vi "OptAcq332Tlog.vi"(0 "Configurations":string[](array[string]), 1 "ConfigsVal In":u16[](array[numeric]), 2 "XY Graph Ref 2":refnum<vi>, 3 "TracerOpts In":u8[](array[numeric]), 4 "AcqenCours":bool caption="Acquisition en Cours", 5 "error in":errorcluster, 6 "VISA Rsrc":refnum<visa-resource-name>="GPIB0::12::INSTR" caption="Nom de la ressource VISA", 7 "Activées In":bool[](array[boolean]) caption="Entrés Activées In") -> (10 "TablesConv":u16[](array[numeric]) caption="No Courbe de conversion" max=60 step=1, 11 "Scan list Out":string[](array[string]), 12 "TracerCourbe":bool[](array[boolean]), 13 "OneChangeAppl":bool caption="Changements Appliqués out", 14 "ConfigsChoisi":string[](array[string]), 15 "ConfigsVal Out":u16[](array[numeric]), 16 "Activées":bool[](array[boolean]) caption="Entrés Activées Out", 17 "TracerOpts Out":u8[](array[numeric]), 18 "Entête":string, 19 "error out":errorcluster)   [LabVIEW 2010]
doc: "Ce Vi permet d'activer et d'attribuer une configuration à chaque entrée du contrôlleur de température. Il permet aussi de choisir les options de traçage des données de température, de niveau d'hélium et de chaufage."
panel:
  in  "Forcer":bool caption="Forcer la mise à jour"
  in  "Chauffage":bool=TRUE caption="Tracer le Chauffage"
  out "Changé":bool[](array[boolean]) caption="Entrés Changé"
  in  "Activé B":bool=TRUE caption="Activée"
  in  "Activé A":bool=TRUE caption="Activée"
  in  "NiveauHe":bool=TRUE caption="Tracer le niveau d'hélium"
  out "LastChangeAppl":bool caption="Changements Appliqués"
  in  "TracerOpt B":u8(ring)=2 caption="Données à Tracer" items=["Unités Capteurs", "Unité Labview", "Ne Pas Tracer"]
  in  "Config B":u16(ring) caption="Nom de la Configuration" items=["Default", "Pompe à adsorption", "Pot à 1K", "Pot à He3", "Échantillon", "Cleaver"]
  in  "TracerOpt A":u8(ring)=2 caption="Données à Tracer" items=["Unités Capteurs", "Unité Labview", "Ne Pas Tracer"]
  in  "Apply":bool
  in  "OK":bool
  in  "Config A":u16(ring) caption="Nom de la Configuration" items=["Default", "Pompe à adsorption", "Pot à 1K", "Pot à He3", "Échantillon", "Cleaver"]
  # "Paramètres d'acquisition"
  # "Entrée A"
  # "Entrée B"
  # "Variables internes"
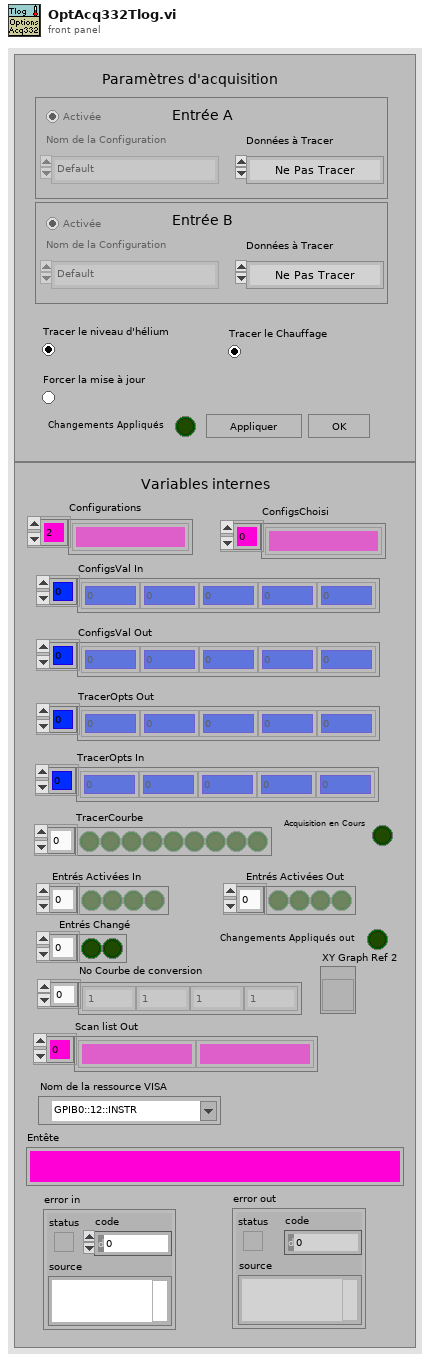
[diagram p1: front panel]
types:
  T1 = enum32{"Invalid", "Standard", "Closed", "Hidden", "Minimized", "Maximized"}
  T2 = typedef "InConfigPar332.ctl" = cluster{"TableTC":u16, "TableConv":u16, "Compensation":u16, "Type":u16}
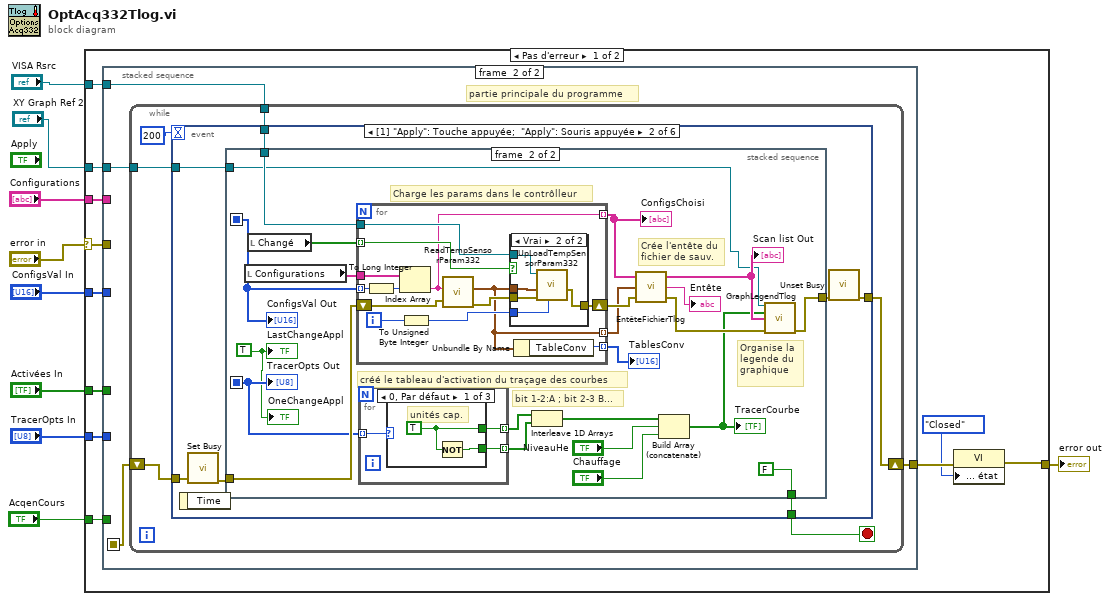
[diagram p0: block diagram]
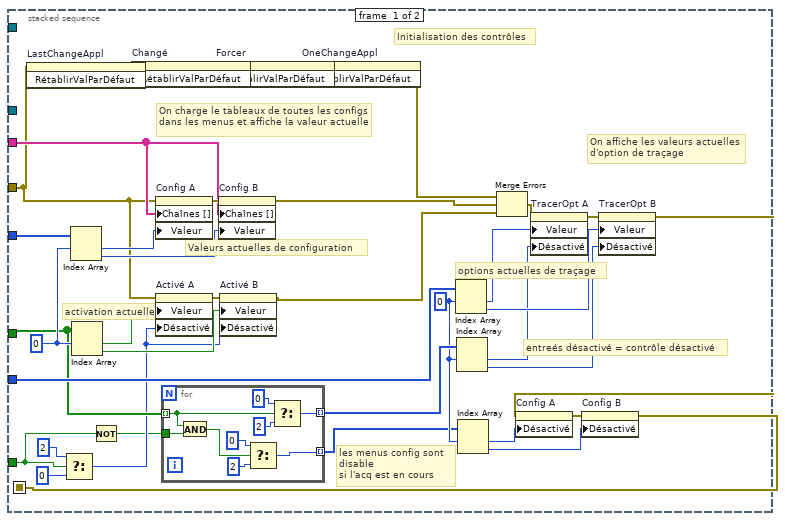
[diagram p2: hidden frame]
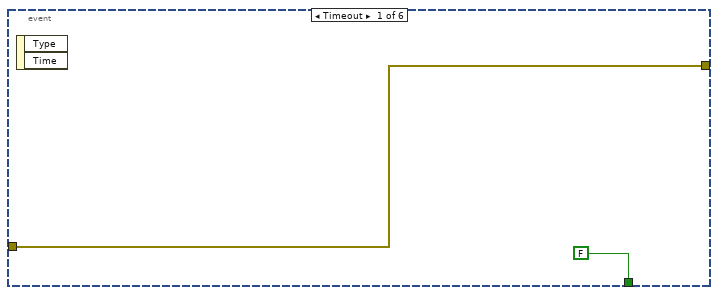
[diagram p3: hidden frame]
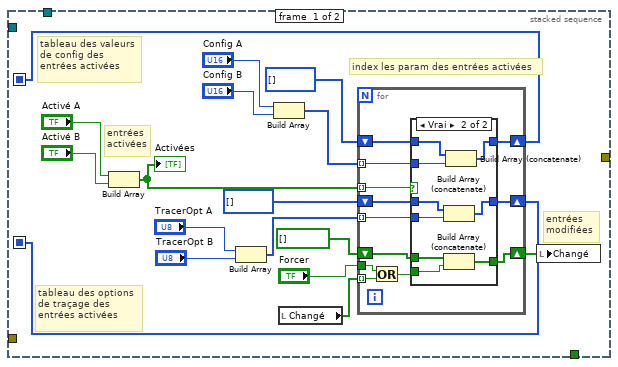
[diagram p4: hidden frame]
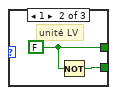
[diagram p6: hidden frame]
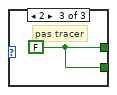
[diagram p7: hidden frame]
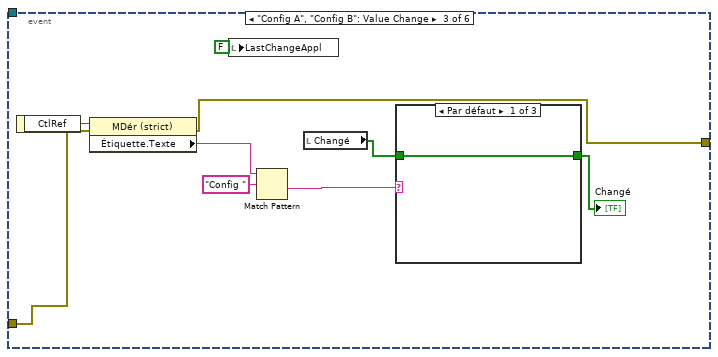
[diagram p9: hidden frame]
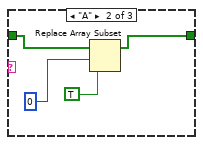
[diagram p10: hidden frame]
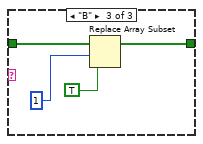
[diagram p11: hidden frame]
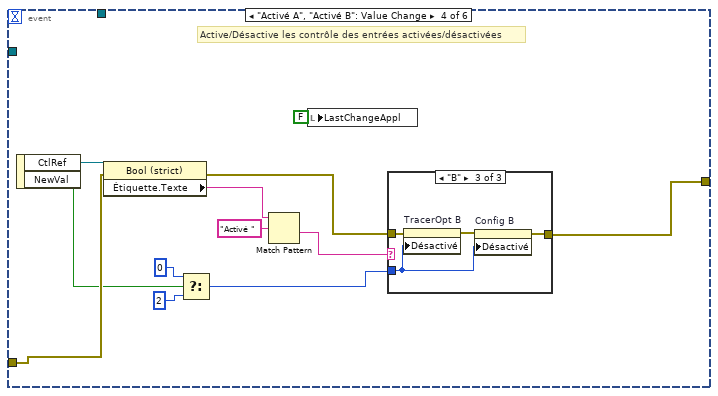
[diagram p12: hidden frame]
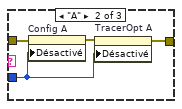
[diagram p14: hidden frame]
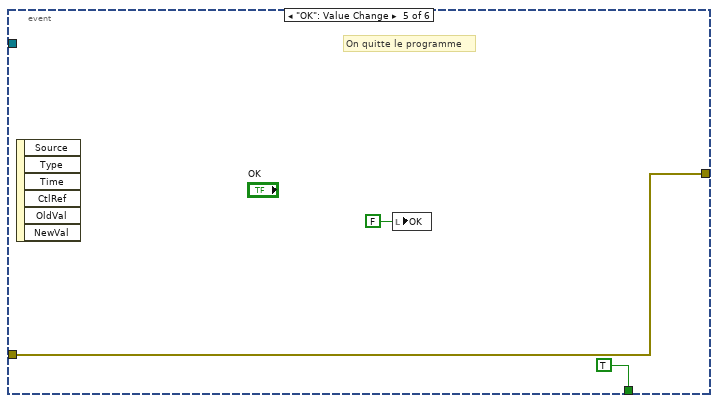
[diagram p15: hidden frame]
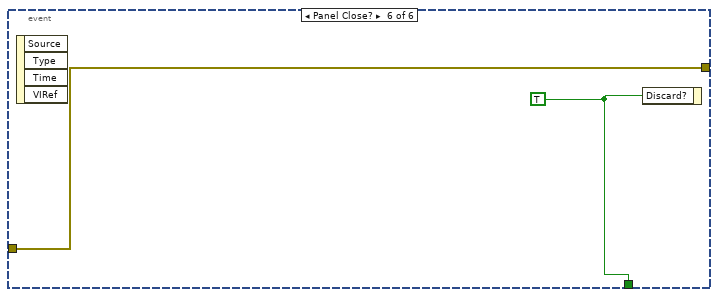
[diagram p16: hidden frame]
diagram:
  n1 = case shown="Pas d'erreur" "error in" {
    selector: "error in" -> [w19 w221]
    tunnel: [w11 w221] -> w9
    tunnel: "Configurations" -> [w20 _]
    tunnel: "ConfigsVal In" -> [w18 _]
    tunnel: "TracerOpts In" -> [w17 _]
    tunnel: "AcqenCours" -> [w16 _]
    tunnel: "Activées In" -> [w15 _]
    tunnel: "XY Graph Ref 2" -> [w14 _]
    tunnel: "VISA Rsrc" -> [w13 _]
    frame No Error {
      n2 = stacked-sequence {
        seq-local: [w21 _] -> [_ w70]
        tunnel: w20 -> [w56 _]
        tunnel: w19 -> [w42 _]
        tunnel: w18 -> [w49 _]
        tunnel: w17 -> [w53 _]
        tunnel: [_ w69] -> w12
        tunnel: w16 -> [w35 _]
        tunnel: w15 -> [w40 _]
        tunnel: w14 -> [_ w68]
        tunnel: w13 -> [_ w67]
        frame #0 {
          w33 = 0 ("index")
          w45 = 0 ("index")
          # "les menus config sont disable\nsi l'acq est en cours"
          # "entreés désactivé = contrôle désactivé"
          # "activation actuelle"
          # "Valeurs actuelles de configuration"
          # "options actuelles de traçage"
          # "On affiche les valeurs actuelles d'option de traçage"
          # "On charge le tableaux de toutes les configs dans les menus et affiche la valeur actuelle"
          # "Initialisation des contrôles"
          n3 = invoke on="LastChangeAppl" class="Bool (strict)" method="RétablirValParDéfaut"(error in=w42) -> (error out=w28:errorcluster)  [unwired: 2 in, 2 out]
          n4 = Select(t=u8 2 ("f"), s=w35, f=u8 0) -> (s? t:f=w39:u8)
          n5 = Index Array(array=w49, index #1=w45) -> (element #1=w55:u16, element #2=w54:u16)  [unwired: 1 in]
          n6 = Index Array(array=w40, index #1=w45) -> (element #1=w44:bool, element #2=w43:bool)  [unwired: 1 in]
          n7 = Not(x=w35) -> (.not. x?=w29:bool)
          n8 = invoke on="Changé" class="Array (strict)" method="RétablirValParDéfaut"(error in=w28) -> (error out=w27:errorcluster)  [unwired: 2 in, 2 out]
          n9 = property on="Config A" class="MDér (strict)"(error in=w42, "Chaînes []"=w56, "Valeur"=w55) -> (error out=w57:errorcluster)  [unwired: 1 in, 1 out]
          n10 = property on="Activé A" class="Bool (strict)"(error in=w42, "Valeur"=w44, "Désactivé"=w39) -> (error out=w41:errorcluster)  [unwired: 1 in, 1 out]
          n11 = for {
            tunnel: w40 -> [w60] mode=indexing
            tunnel: [w62] -> w38 mode=indexing
            tunnel: w29 -> [w59]
            tunnel: [w61] -> w30 mode=indexing
            n12 = And(x=w60, y=w59) -> (x .and. y?=w58:bool)
            n13 = Select(t=u8 0 ("f"), s=w58, f=u8 2) -> (s? t:f=w61:u8)
            n14 = Select(t=u8 0 ("f"), s=w60, f=u8 2) -> (s? t:f=w62:u8)
          }
          n15 = invoke on="Forcer" class="Boolean (strict)" method="RétablirValParDéfaut"(error in=w27) -> (error out=w26:errorcluster)  [unwired: 2 in, 2 out]
          n16 = property on="Config B" class="MDér (strict)"(error in=w57, "Chaînes []"=w56, "Valeur"=w54) -> (error out=w23:errorcluster)  [unwired: 1 in, 1 out]
          n17 = property on="Activé B" class="Bool (strict)"(error in=w41, "Valeur"=w43, "Désactivé"=w39) -> (error out=w24:errorcluster)  [unwired: 1 in, 1 out]
          n18 = invoke on="OneChangeAppl" class="Boolean (strict)" method="RétablirValParDéfaut"(error in=w26) -> (error out=w25:errorcluster)  [unwired: 2 in, 2 out]
          n19 = Index Array(array=w53, index #1=w33) -> (element #1=w51:u8, element #2=w50:u8)  [unwired: 1 in]
          n20 = Index Array(array=w38, index #1=w33) -> (element #1=w37:u8, element #2=w36:u8)  [unwired: 1 in]
          n21 = Index Array(array=w30, index #1=w33) -> (element #1=w32:u8, element #2=w31:u8)  [unwired: 1 in]
          n22 = Merge Errors(w25, w23, w24) -> (w47:errorcluster)
          n23 = property on="TracerOpt A" class="MDér (strict)"(error in=w47, "Valeur"=w51, "Désactivé"=w37) -> (error out=w52:errorcluster)  [unwired: 1 in, 1 out]
          n24 = property on="TracerOpt B" class="MDér (strict)"(error in=w52, "Valeur"=w50, "Désactivé"=w36) -> (error out=w22:errorcluster)  [unwired: 1 in, 1 out]
          n25 = property on="Config A" class="MDér (strict)"(error in=w22, "Désactivé"=w32) -> (error out=w34:errorcluster)  [unwired: 1 in, 1 out]
          n26 = property on="Config B" class="MDér (strict)"(error in=w34, "Désactivé"=w31) -> (error out=w21:errorcluster)  [unwired: 1 in, 1 out]
        }
        frame #1 {
          # "partie principale du programme"
          n27 = while {
            shift-right: [w73] -> w69
            shift-left: w70 -> [w75]
            tunnel: w68 -> [w72]
            tunnel: w67 -> [w71]
            stop <- w74 stop-if-true
            n28 = event shown="[1] \"Apply\": Touche appuyée;  \"Apply\": Souris appuyée" {
              selector: _ -> [_ _ _ _ _ _]
              dyn-events: _ -> [_ _ _ _ _ _]
              timeout: 200 -> [_ _ _ _ _ _]
              tunnel: w75 -> [w77 w83 w182 w205 w218 w219]
              tunnel: [w77 w81 w178 w201 w218 w219] -> w73
              tunnel: [FALSE w85 _ _ TRUE w220] -> w74
              tunnel: w72 -> [_ w84 _ _ _ _]
              tunnel: w71 -> [_ w79 _ _ _ _]
              event Timeout {
                n29 = event-data() -> ()  [unwired: 1 in, 2 out]
              }
              event "Apply": Key Down; "Apply": Mouse Down {
                n30 = event-data() -> ()  [unwired: 1 in, 1 out]
                n31 = call <vilib>:"Set Busy.vi"("error in (no error)"=w83) -> ("error out"=w82:errorcluster)  [unwired: 9 in, 1 out]
                n32 = stacked-sequence {
                  seq-local: [w94 _] -> [_ w142]
                  seq-local: [w95 _] -> [_ w143]
                  tunnel: w82 -> [_ w149]
                  tunnel: [_ w134] -> w80
                  tunnel: [_ FALSE] -> w85
                  tunnel: w84 -> [_ w127]
                  tunnel: w79 -> [_ w131]
                  frame #0 {
                    # "entrées\nmodifiées"
                    # "entrées\nactivées"
                    # "tableau des options\nde traçage des \nentrées activées"
                    # "tableau des valeurs\nde config des \nentrées activées"
                    # "index les param des entrées activées"
                    n33 = Build Array("Activé A", "Activé B") -> (w93:bool[])
                    "Activées" <- w93
                    n34 = Build Array("TracerOpt A", "TracerOpt B") -> (w98:u8[])
                    n35 = Build Array("Config A", "Config B") -> (w99:u16[])
                    n36 = local read "Changé"() -> (w90:bool[])
                    n37 = for {
                      tunnel: w99 -> [w114] mode=indexing
                      tunnel: w98 -> [w113] mode=indexing
                      shift-right: [w111] -> w94
                      shift-left: u16[] [] -> [w112]
                      shift-right: [w109] -> w95
                      shift-left: u8[] [] -> [w110]
                      tunnel: w93 -> [w106] mode=indexing
                      tunnel: w90 -> [w105] mode=indexing
                      shift-right: [w108] -> w89
                      shift-left: bool[] [] -> [w107]
                      tunnel: "Forcer" -> [w104]
                      n38 = Or(x=w104, y=w105) -> (x .or. y?=w103:bool)
                      n39 = case shown="Vrai" w106 {
                        tunnel: w114 -> [_ w126]
                        tunnel: w113 -> [_ w123]
                        tunnel: w112 -> [w117 w125]
                        tunnel: [w117 w124] -> w111
                        tunnel: w110 -> [w116 w122]
                        tunnel: [w116 w121] -> w109
                        tunnel: w103 -> [_ w118]
                        tunnel: [w115 w120] -> w108
                        tunnel: w107 -> [w115 w119]
                        frame False {
                        }
                        frame True {
                          n40 = Build Array (concatenate)(w122, w123) -> (w121:u8[])
                          n41 = Build Array (concatenate)(w119, w118) -> (w120:bool[])
                          n42 = Build Array (concatenate)(w125, w126) -> (w124:u16[])
                        }
                      }
                    }
                    n43 = local write "Changé"(w89) -> ()
                  }
                  frame #1 {
                    w128 = TRUE
                    # "Charge les params dans le contrôlleur"
                    # "Organise la\nlegende du \ngraphique"
                    # "bit 1-2:A ; bit 2-3 B..."
                    # "créé le tableau d'activation du traçage des courbes"
                    # "Crée l'entête du fichier de sauv."
                    n44 = local read "Configurations"() -> (w144:string[])
                    n45 = local read "Changé"() -> (w132:bool[])
                    n46 = for {
                      tunnel: w144 -> [w170]
                      tunnel: [w159] -> w137 mode=indexing
                      shift-right: [w167] -> w147
                      shift-left: w149 -> [w164]
                      tunnel: w142 -> [w166] mode=indexing
                      tunnel: [w165] -> w141 mode=indexing
                      tunnel: [w158] -> w133 mode=indexing
                      tunnel: w132 -> [w161] mode=indexing
                      tunnel: w131 -> [w160]
                      i -> [w168]
                      n47 = To Long Integer(number=w166) -> (32bit integer=w169:i32)
                      n48 = Index Array(array=w170, index=w169) -> (element=w159:string)
                      n49 = To Unsigned Byte Integer(number=w168) -> (unsigned 8bit integer=w162:u8)
                      n50 = call <userlib>:"ReadTempSensorParam332.vi"("Nom"=w159, "Error in"=w164) -> ("SensorPar"=w158:T2, "Error out"=w163:errorcluster)  [unwired: 1 in, 1 out]
                      n51 = case shown="Vrai" w161 {
                        tunnel: w162 -> [_ w172]
                        tunnel: [w171 w176] -> w167
                        tunnel: w163 -> [w171 w175]
                        tunnel: w158 -> [_ w174]
                        tunnel: w160 -> [_ w173]
                        frame False {
                        }
                        frame True {
                          n52 = call <userlib>:"UpLoadTempSensorParam332.vi"("Input"=w172, "Error in"=w175, "SensorParIn"=w174, "VISA Rsrc"=w173) -> ("Error out"=w176:errorcluster)  [unwired: 4 in, 1 out]
                        }
                      }
                      n53 = Unbundle By Name(w158) -> ("TableConv"=w165:u16)
                    }
                    "ConfigsChoisi" <- w137
                    "TablesConv" <- w141
                    n54 = for {
                      tunnel: w143 -> [w152] mode=indexing
                      tunnel: [w151] -> w140 mode=indexing
                      tunnel: [w150] -> w139 mode=indexing
                      n55 = case shown="0, Par défaut" w152 {
                        tunnel: [w154 w156 w157] -> w151
                        tunnel: [w153 w155 w157] -> w150
                        frame 0, Default {
                          w154 = TRUE
                          # "unités cap."
                          n56 = Not(x=w154) -> (.not. x?=w153:bool)
                        }
                        frame 1 {
                          w156 = FALSE
                          # "unité LV"
                          n57 = Not(x=w156) -> (.not. x?=w155:bool)
                        }
                        frame 2 {
                          w157 = FALSE
                          # "pas tracer"
                        }
                      }
                    }
                    n58 = Interleave 1D Arrays(w140, w139) -> (w138:bool[])
                    n59 = call <userlib>:"EntêteFichierTlog.vi"("Error in"=w147, "TSensPAr"=w133, "ConfigChoisies"=w137) -> ("error out"=w136:errorcluster, "Entête"=→"Entête":string, "Scan list Out"=w135:string[])
                    "Scan list Out" <- w135
                    n60 = Build Array (concatenate)(w138, "NiveauHe", "Chauffage") -> (w129:bool[])
                    "TracerCourbe" <- w129
                    n61 = call <userlib>:"GraphLegendTlog.vi"("XY Graph Ref"=w127, "TracerCourbe"=w129, "Scan list"=w135, "error in (no error)"=w136) -> ("error out"=w134:errorcluster)  [unwired: 11 in]
                    "LastChangeAppl" <- w128
                    "ConfigsVal Out" <- w142
                    "TracerOpts Out" <- w143
                    "OneChangeAppl" <- w128
                  }
                }
                n62 = call <vilib>:"Unset Busy.vi"("error in (no error)"=w80) -> ("error out"=w81:errorcluster)  [unwired: 10 in]
              }
              event "Config A", "Config B": Value Change {
                n63 = event-data() -> ("CtlRef"=w183:refnum<vi>)  [unwired: 1 in]
                n64 = property class="MDér (strict)"(reference=w183, error in=w182) -> (error out=w178:errorcluster, "Étiquette.Texte"=w184:string)  [unwired: 1 out]
                n65 = local write "LastChangeAppl"(FALSE ("ChangeAppl")) -> ()
                n66 = Match Pattern(string=w184, regular expression="Config ") -> (after substring=w181:string)  [unwired: 1 in, 3 out]
                n67 = local read "Changé"() -> (w180:bool[])
                n68 = case shown="Par défaut" w181 {
                  tunnel: w180 -> [w186 w188 w193]
                  tunnel: [w186 w187 w191] -> w179
                  frame Default {
                  }
                  frame "A" {
                    n69 = Replace Array Subset(array=w188, new element=TRUE, index=0) -> (w187:bool[])
                  }
                  frame "B" {
                    n70 = Replace Array Subset(array=w193, new element=TRUE, index=1) -> (w191:bool[])
                  }
                }
                "Changé" <- w179
              }
              event "Activé A", "Activé B": Value Change {
                # "Active/Désactive les contrôle des entrées activées/désactivées"
                n71 = event-data() -> ("CtlRef"=w206:refnum<vi>, "NewVal"=w198:bool)  [unwired: 1 in]
                n72 = property class="Bool (strict)"(reference=w206, error in=w205) -> (error out=w202:errorcluster, "Étiquette.Texte"=w203:string)  [unwired: 1 out]
                n73 = Select(t=u8 0 ("f"), s=w198, f=u8 2) -> (s? t:f=w197:u8)
                n74 = Match Pattern(string=w203, regular expression="Activé ") -> (after substring=w196:string)  [unwired: 1 in, 3 out]
                n75 = local write "LastChangeAppl"(FALSE ("ChangeAppl")) -> ()
                n76 = case shown="\"B\"" w196 {
                  tunnel: w202 -> [w207 w211 w213]
                  tunnel: [w207 w209 w215] -> w201
                  tunnel: w197 -> [_ w208 w212]
                  frame Default {
                  }
                  frame "A" {
                    n77 = property on="Config A" class="MDér (strict)"(error in=w211, "Désactivé"=w208) -> (error out=w210:errorcluster)  [unwired: 1 in, 1 out]
                    n78 = property on="TracerOpt A" class="MDér (strict)"(error in=w210, "Désactivé"=w208) -> (error out=w209:errorcluster)  [unwired: 1 in, 1 out]
                  }
                  frame "B" {
                    n79 = property on="TracerOpt B" class="MDér (strict)"(error in=w213, "Désactivé"=w212) -> (error out=w214:errorcluster)  [unwired: 1 in, 1 out]
                    n80 = property on="Config B" class="MDér (strict)"(error in=w214, "Désactivé"=w212) -> (error out=w215:errorcluster)  [unwired: 1 in, 1 out]
                  }
                }
              }
              event "OK": Value Change {
                # "On quitte le programme"
                n81 = event-data() -> ()  [unwired: 1 in, 6 out]
                n82 = local write "OK"(FALSE ("OK")) -> ()
              }
              event Panel Close? {
                w220 = TRUE ("Discard?")
                n83 = event-data() -> ()  [unwired: 1 in, 4 out]
                n84 = event-data("Discard?"=w220) -> ()  [unwired: 1 in, 1 out]
              }
            }
          }
        }
      }
      n85 = property class="VI"(error in=w12, "Fenêtre face-avant : état"=T1."Closed" ("Front Panel Window:State")) -> (error out=w11:errorcluster)  [unwired: 1 in, 1 out]
    }
    frame Error {
    }
  }
  "error out" <- w9
